vi "Using shift registers to save data.vi"() -> ()   [LabVIEW 2018]
panel:
  out "Waveform Chart":waveform(dbl)(graph)
  in  "stop":bool
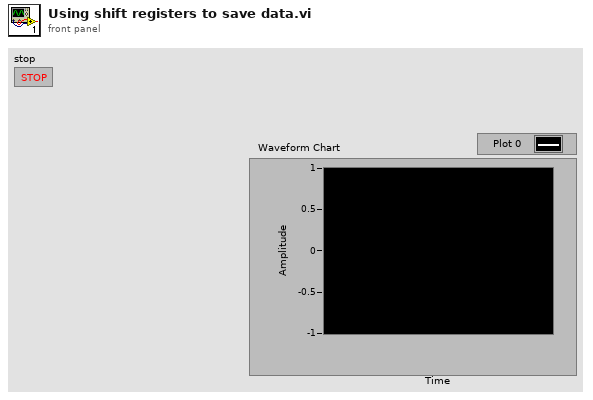
[diagram p1: front panel]
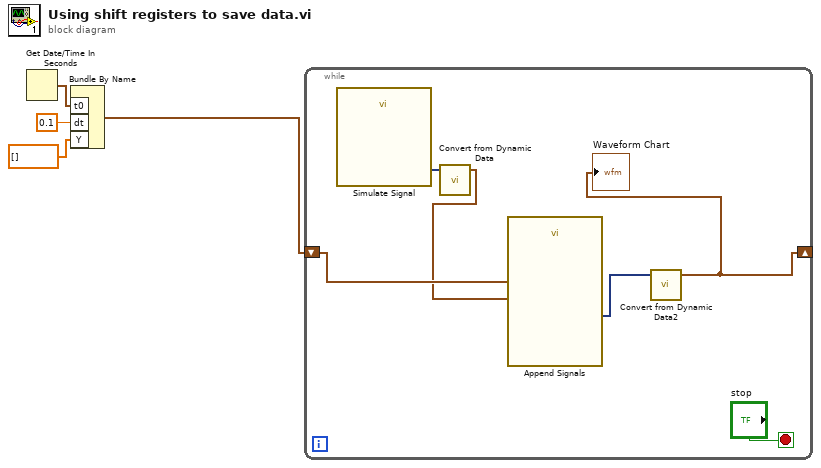
[diagram p0: block diagram]
diagram:
  n1 = Get Date/Time In Seconds() -> (seconds since 1Jan1904=w4:timestamp)
  n2 = Bundle By Name("t0"=w4, "dt"=0.1, "Y"=dbl[] []) -> (w1:waveform(dbl))  [unwired: 1 in]
  n3 = while {
    shift-right: [w5] -> _
    shift-left: w1 -> [w8]
    stop <- "stop" stop-if-true
    n4 = call "Simulate Signal"() -> ("Sine"=w9:dynamicdata)  [unwired: 14 in, 1 out]
    n5 = call "Convert from Dynamic Data"("Dynamic Data Type"=w9) -> ("Waveform"=w7:waveform(dbl))  [unwired: 3 in]
    n6 = call "Append Signals"("Input Signal B"=w7, "Input Signal A"=w8) -> ("Appended Signals"=w6:dynamicdata)  [unwired: 8 in, 1 out]
    n7 = call "Convert from Dynamic Data2"("Dynamic Data Type"=w6) -> ("Waveform"=w5:waveform(dbl))  [unwired: 3 in]
    "Waveform Chart" <- w5
  }
